vi "ArticulateAutonDrive.vi"(4 "Stop Time":dbl, 6 "Drive Time":dbl, 7 "Right Input":dbl format="%#_13g", 9 "Left Input":dbl format="%#_13g", 10 "POV Input_2":i32=-1, 11 "POV Input_1":i32=-1) -> ()   [LabVIEW 2015]
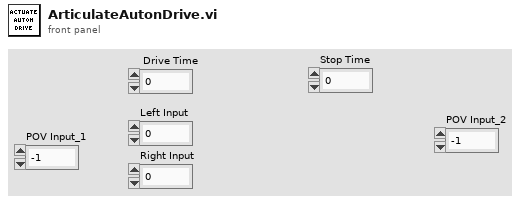
[diagram p1: front panel]
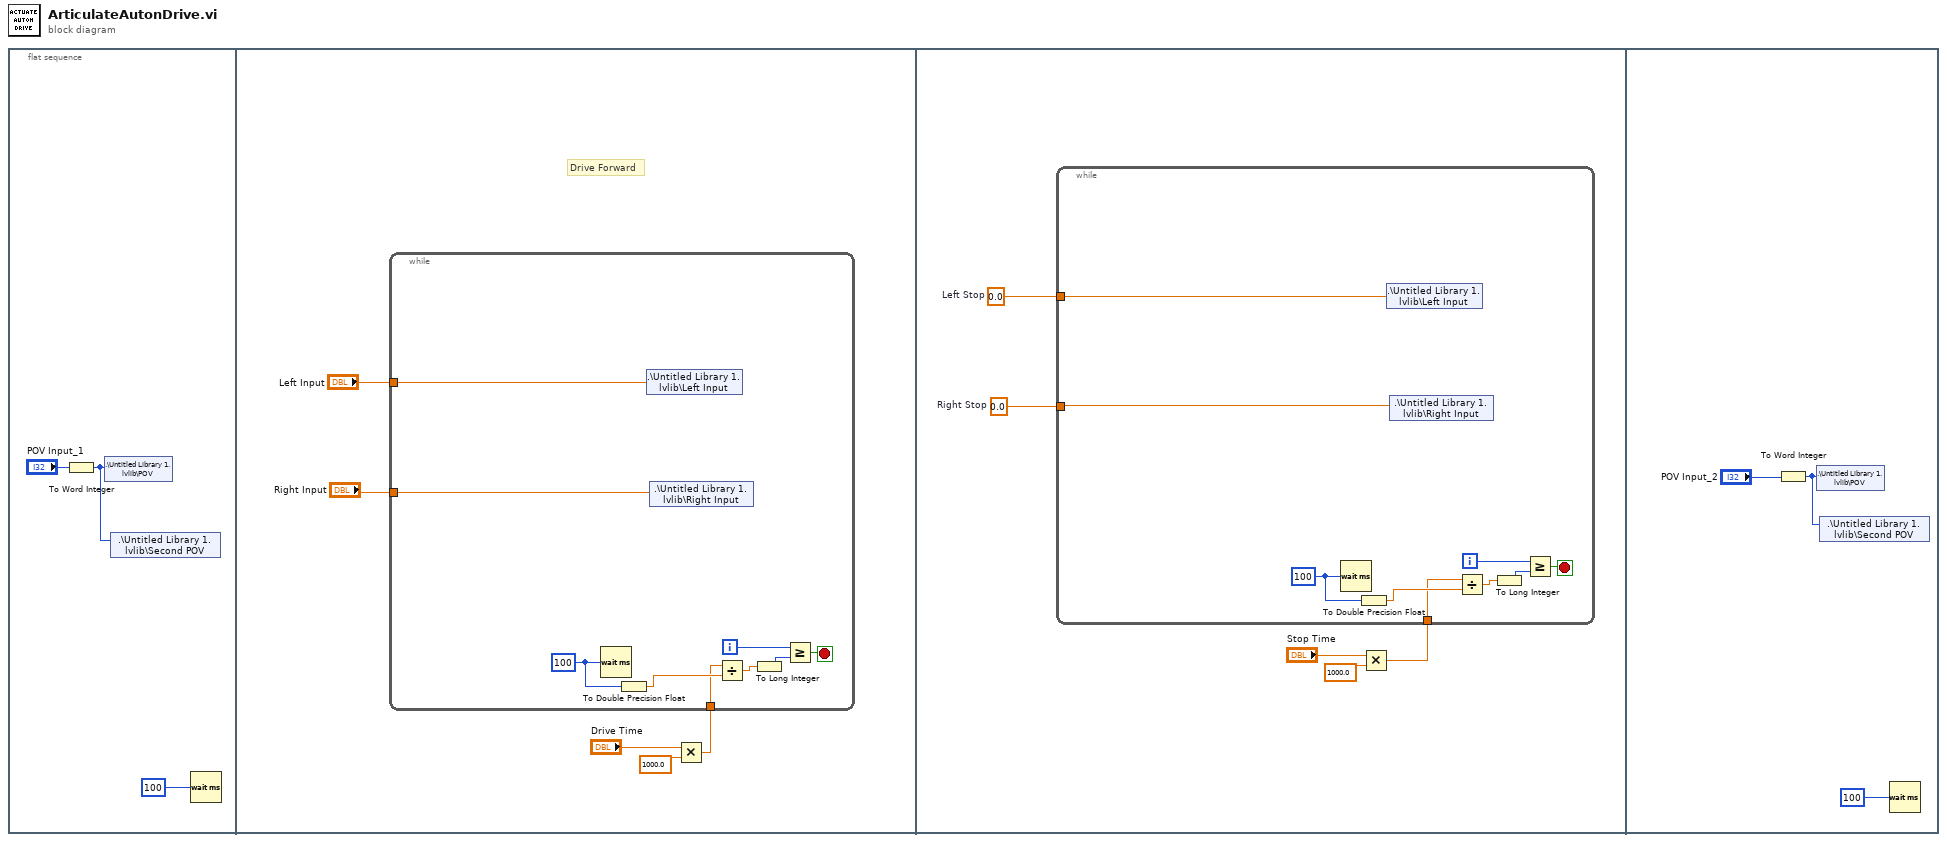
[diagram p0: block diagram]
diagram:
  n1 = flat-sequence {
    frame #0 {
      n2 = To Word Integer(number="POV Input_1") -> (16bit integer=w1:i16)
      n3 = shared-variable ".\\Untitled Library 1.lvlib\\POV"(w1) -> ()  [unwired: 1 in, 1 out]
      n4 = shared-variable ".\\Untitled Library 1.lvlib\\Second POV"(w1) -> ()  [unwired: 1 in, 1 out]
      n5 = Wait (ms)(milliseconds to wait=u32 100) -> ()  [unwired: 1 out]
    }
    frame #1 {
      # "Drive Forward"
      n6 = Multiply(x="Drive Time", y=1000.0) -> (x*y=w8:dbl)
      n7 = while {
        tunnel: "Left Input" -> [w10]
        tunnel: "Right Input" -> [w9]
        tunnel: w8 -> [w11]
        i -> [w13]
        stop <- w12 stop-if-true
        w17 = u32 100 ("milliseconds to wait")
        n8 = Wait (ms)(milliseconds to wait=w17) -> ()  [unwired: 1 out]
        n9 = To Double Precision Float(number=w17) -> (double precision float=w16:dbl)
        n10 = shared-variable ".\\Untitled Library 1.lvlib\\Left Input"(w10) -> ()  [unwired: 1 in, 1 out]
        n11 = shared-variable ".\\Untitled Library 1.lvlib\\Right Input"(w9) -> ()  [unwired: 1 in, 1 out]
        n12 = Divide(x=w11, y=w16) -> (x/y=w15:dbl)
        n13 = To Long Integer(number=w15) -> (32bit integer=w14:i32)
        n14 = Greater Or Equal?(x=w13, y=w14) -> (x >= y?=w12:bool)
      }
    }
    frame #2 {
      w21 = 0.0  # Right Stop
      w22 = 0.0  # Left Stop
      n15 = Multiply(x="Stop Time", y=1000.0) -> (x*y=w18:dbl)
      n16 = while {
        tunnel: w22 -> [w24]
        tunnel: w21 -> [w23]
        tunnel: w18 -> [w25]
        i -> [w27]
        stop <- w26 stop-if-true
        w31 = u32 100 ("milliseconds to wait")
        n17 = Wait (ms)(milliseconds to wait=w31) -> ()  [unwired: 1 out]
        n18 = To Double Precision Float(number=w31) -> (double precision float=w30:dbl)
        n19 = shared-variable ".\\Untitled Library 1.lvlib\\Left Input"(w24) -> ()  [unwired: 1 in, 1 out]
        n20 = shared-variable ".\\Untitled Library 1.lvlib\\Right Input"(w23) -> ()  [unwired: 1 in, 1 out]
        n21 = Divide(x=w25, y=w30) -> (x/y=w29:dbl)
        n22 = To Long Integer(number=w29) -> (32bit integer=w28:i32)
        n23 = Greater Or Equal?(x=w27, y=w28) -> (x >= y?=w26:bool)
      }
    }
    frame #3 {
      n24 = To Word Integer(number="POV Input_2") -> (16bit integer=w33:i16)
      n25 = shared-variable ".\\Untitled Library 1.lvlib\\POV"(w33) -> ()  [unwired: 1 in, 1 out]
      n26 = shared-variable ".\\Untitled Library 1.lvlib\\Second POV"(w33) -> ()  [unwired: 1 in, 1 out]
      n27 = Wait (ms)(milliseconds to wait=u32 100) -> ()  [unwired: 1 out]
    }
  }
